vi "Functions.vi"(10 "FUNCTION":string, 11 "StackIn":dbl[](array[numeric])) -> (3 "StackOut":dbl[](array[numeric]))   [LabVIEW 2019, in "Eval.lvlib"]
uses:
  Eval.lvlib
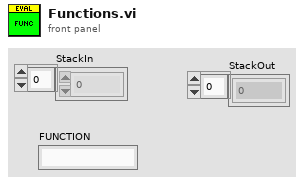
[diagram p1: front panel]
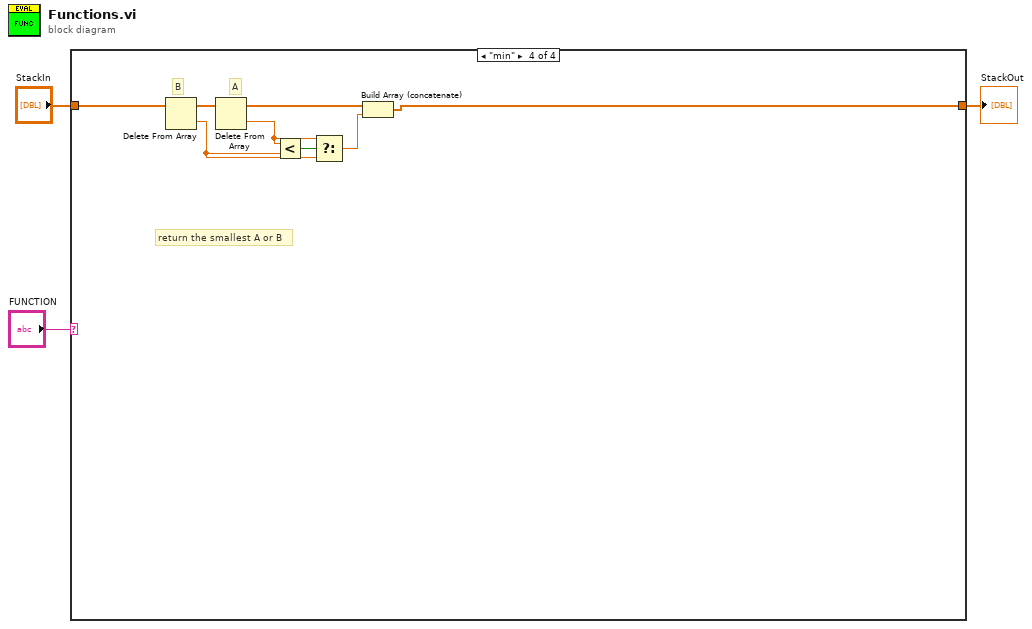
[diagram p0: block diagram]
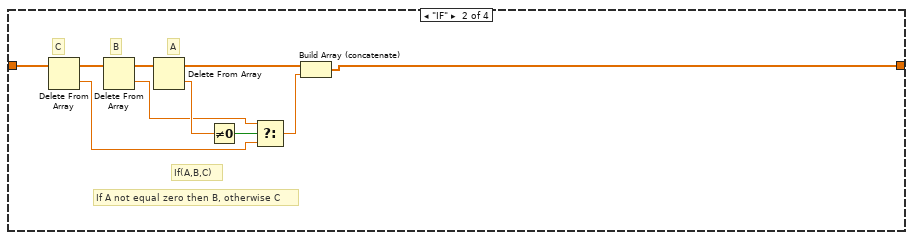
[diagram p3: hidden frame]
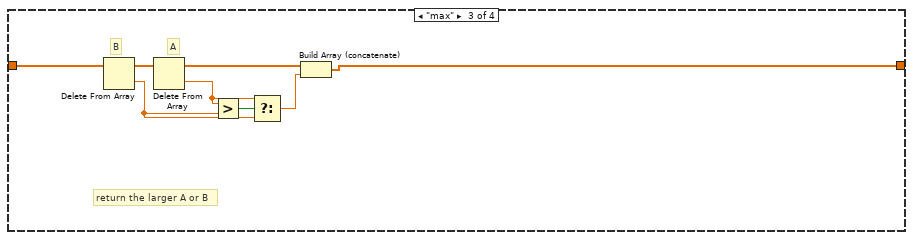
[diagram p4: hidden frame]
diagram:
  n1 = case shown="\"min\"" "FUNCTION" {
    tunnel: "StackIn" -> [w4 w14 w19 w27]
    tunnel: [w4 w5 w20 w28] -> w2
    frame "False", Default {
      # "Do nothing"
    }
    frame "IF" {
      # "C"
      # "B"
      # "A"
      # "If A not equal zero then B, otherwise C"
      # "If(A,B,C)"
      n2 = Delete From Array(array=w14) -> (deleted portion=w8:dbl, array with subset deleted=w13:dbl[])  [unwired: 2 in]
      n3 = Delete From Array(array=w13) -> (deleted portion=w9:dbl, array with subset deleted=w12:dbl[])  [unwired: 2 in]
      n4 = Delete From Array(array=w12) -> (deleted portion=w11:dbl, array with subset deleted=w7:dbl[])  [unwired: 2 in]
      n5 = Not Equal To 0?(x=w11) -> (x != 0?=w10:bool)
      n6 = Select(t=w9, s=w10, f=w8) -> (s? t:f=w6:dbl)
      n7 = Build Array (concatenate)(w7, w6) -> (w5:dbl[])
    }
    frame "max" {
      # "B"
      # "A"
      # "return the larger A or B"
      n8 = Delete From Array(array=w19) -> (deleted portion=w16:dbl, array with subset deleted=w22:dbl[])  [unwired: 2 in]
      n9 = Delete From Array(array=w22) -> (deleted portion=w17:dbl, array with subset deleted=w21:dbl[])  [unwired: 2 in]
      n10 = Greater?(x=w17, y=w16) -> (0:w18:bool)
      n11 = Select(t=w17, s=w18, f=w16) -> (s? t:f=w15:dbl)
      n12 = Build Array (concatenate)(w21, w15) -> (w20:dbl[])
    }
    frame "min" {
      # "B"
      # "A"
      # "return the smallest A or B"
      n13 = Delete From Array(array=w27) -> (deleted portion=w24:dbl, array with subset deleted=w30:dbl[])  [unwired: 2 in]
      n14 = Delete From Array(array=w30) -> (deleted portion=w25:dbl, array with subset deleted=w29:dbl[])  [unwired: 2 in]
      n15 = Less?(x=w25, y=w24) -> (x < y?=w26:bool)
      n16 = Select(t=w25, s=w26, f=w24) -> (s? t:f=w23:dbl)
      n17 = Build Array (concatenate)(w29, w23) -> (w28:dbl[])
    }
  }
  "StackOut" <- w2
